vi "Untitled 1.vi"() -> ()   [LabVIEW 2020]
panel:
  in  "InC":dbl
  out "Out":dbl
  in  "InB":dbl
  in  "InA":dbl
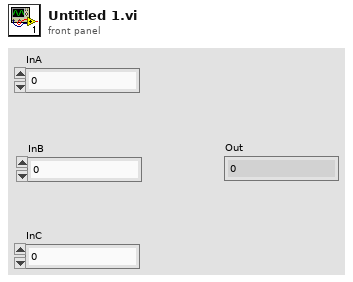
[diagram p1: front panel]
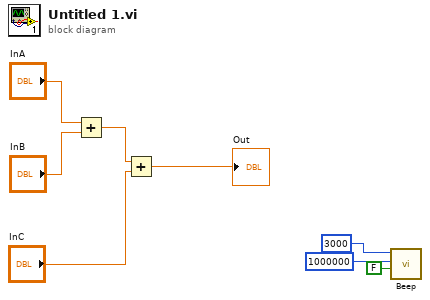
[diagram p0: block diagram]
diagram:
  n1 = Add(x="InA", y="InB") -> (x+y=w6:dbl)
  n2 = Add(x=w6, y="InC") -> (x+y=→"Out":dbl)
  n3 = call <vilib>:"Beep.vi"("use system alert? (T)"=FALSE, "duration (msec)"=u32 1000000, "frequency (Hz)"=u32 3000) -> ()  [unwired: 9 in]
